vi "Write UpdatedValues.vi"(8 "error in (no error)":errorcluster, 10 "UpdatedValues":bool, 11 "VariableManager in":refnum<class "VariableManager.lvclass">) -> (0 "error out":errorcluster, 3 "VariableManager out":refnum<class "VariableManager.lvclass">)   [LabVIEW 2013, in "VariableManager.lvclass"]
uses:
  VariableManager.lvclass
  VariableManager.lvclass/VariableManager.ctl
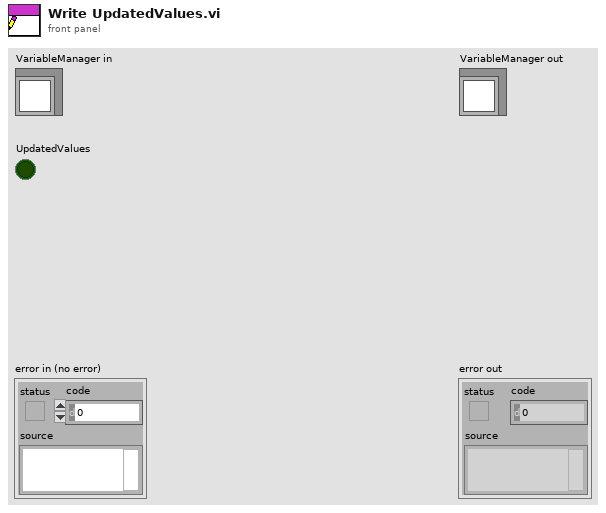
[diagram p1: front panel]
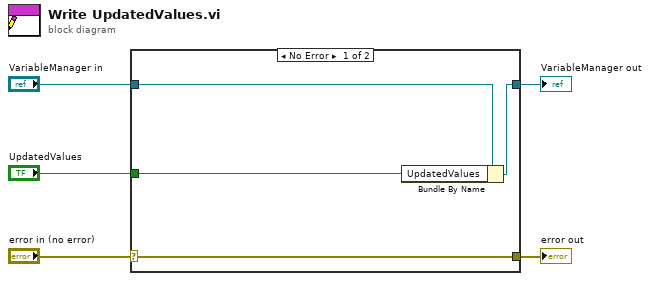
[diagram p0: block diagram]
diagram:
  n1 = case shown="No Error" "error in (no error)" {
    selector: "error in (no error)" -> [w9 w10]
    tunnel: [w9 w10] -> w4
    tunnel: [w7 w11] -> w2
    tunnel: "VariableManager in" -> [w8 w11]
    tunnel: "UpdatedValues" -> [w6 _]
    frame No Error {
      n2 = Bundle By Name(cluster=w8, "UpdatedValues"=w6) -> (w7:refnum<class "VariableManager.lvclass">)
    }
    frame Error {
    }
  }
  "error out" <- w4
  "VariableManager out" <- w2
